vi "Сортирова.vi"() -> ()   [LabVIEW 2013]
panel:
  out "Array 2":dbl[](array[numeric])
  out "Array":dbl[](array[numeric])
  in  "кол-во":i32=10
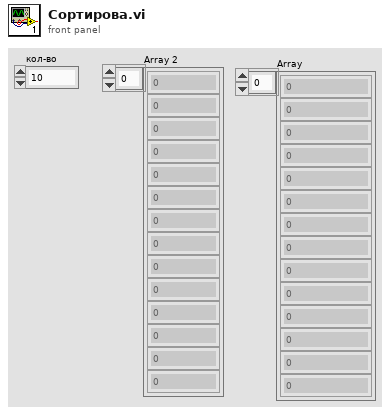
[diagram p1: front panel]
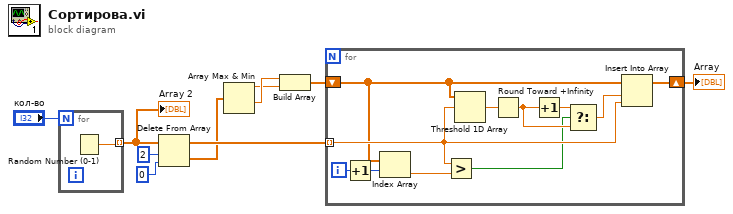
[diagram p0: block diagram]
diagram:
  n1 = for {
    N: "кол-во" -> [_]
    tunnel: [w11] -> w1 mode=indexing
    n2 = Random Number (0-1)() -> (number: 0 to 1=w11:dbl)
  }
  "Array 2" <- w1
  n3 = Delete From Array(array=w1, length=2, index=0) -> (deleted portion=w6:dbl[], array with subset deleted=w7:dbl[])
  n4 = Array Max & Min(array=w6) -> (max value=w2:dbl, min value=w5:dbl)  [unwired: 2 out]
  n5 = Build Array(w5, w2) -> (w9:dbl[])
  n6 = for {
    tunnel: w7 -> [w20] mode=indexing
    shift-right: [w21] -> w4
    shift-left: w9 -> [w14]
    i -> [w15]
    n7 = Increment(x=w15) -> (x+1=w13:i32)
    n8 = Index Array(array=w14, index=w13) -> (element=w12:dbl)
    n9 = Greater?(x=w20, y=w12) -> (0:w16:bool)
    n10 = Threshold 1D Array(2:w20, 3:w14) -> (0:w22:dbl)  [unwired: 1 in]
    n11 = Round Toward +Infinity(x=w22) -> (ceil(x): smallest int >= x=w18:dbl)
    n12 = Increment(x=w18) -> (x+1=w19:dbl)
    n13 = Select(t=w19, s=w16, f=w18) -> (s? t:f=w17:dbl)
    n14 = Insert Into Array(array=w14, index=w17, new element=w20) -> (w21:dbl[])
  }
  "Array" <- w4
